vi "Game.vi"() -> ()   [LabVIEW 2012]
uses:
  <vilib>/Analysis/3filter.llb/Filter Passband Type.ctl
  Class/LV Wiimote Interface.lvclass
  <vilib>/ptbypt/NI_PtbyPt.lvlib
  <vilib>/Analysis/NI_AALBase.lvlib
panel:
  out "actual loop rate (ms)":u32
  in  "order":i32=2
  out "error":i32
  out "Waveform Chart":cluster{"X":sgl, "Filtered x":dbl}(graph)
  in  "low cutoff freq: fl":dbl=0.125 format="%0.3f"
  in  "Loop Rate":u32=50
  in  "high cutoff freq: fh":dbl=0.45000000000000007 format="%0.3f"
  in  "stop":bool
  in  "X, Y or Z":i32
  out "error out":errorcluster
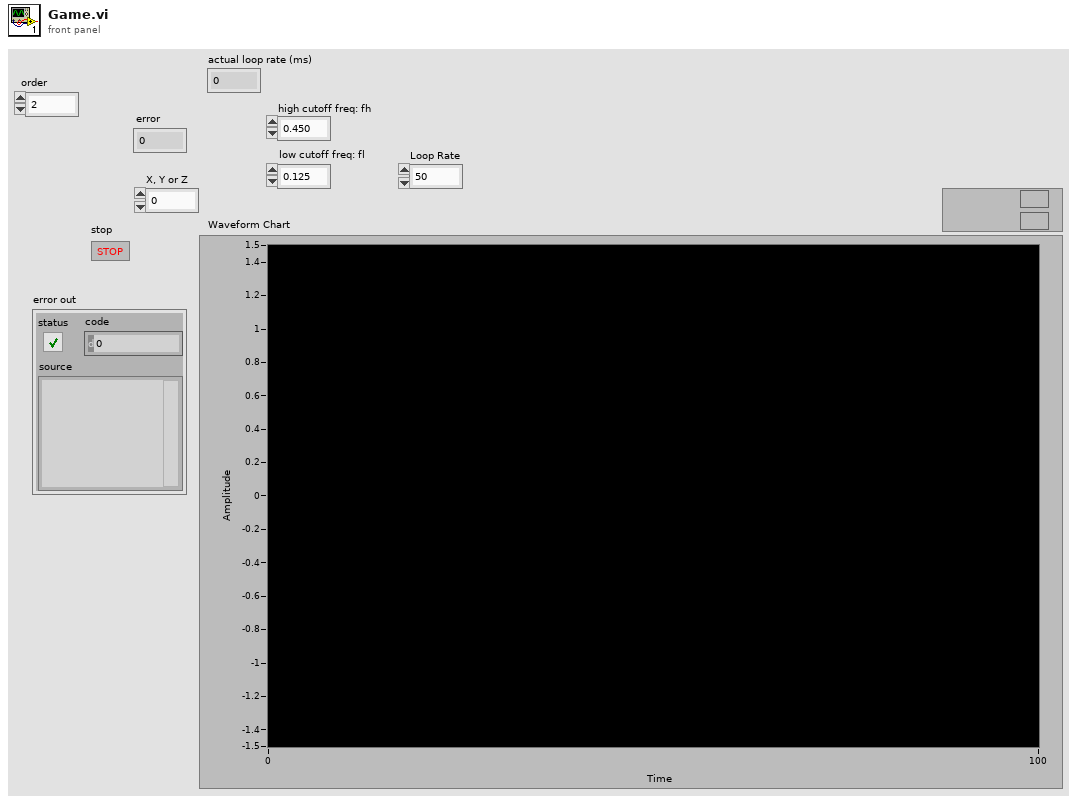
[diagram p1: front panel]
types:
  T1 = typedef "LV Wiimote Interface.ctl" = refnum<class "LV Wiimote Interface.lvclass">
  T2 = typedef "NI_AALBase.lvlib/Filter Passband Type.ctl" = enum32{"Lowpass", "Highpass", "Bandpass", "Bandstop"}
  T3 = typedef "LV Wiimote Interface.lvclass/XYZ Acceleration.ctl" = cluster{"X":sgl, "Y":sgl, "Z":sgl}
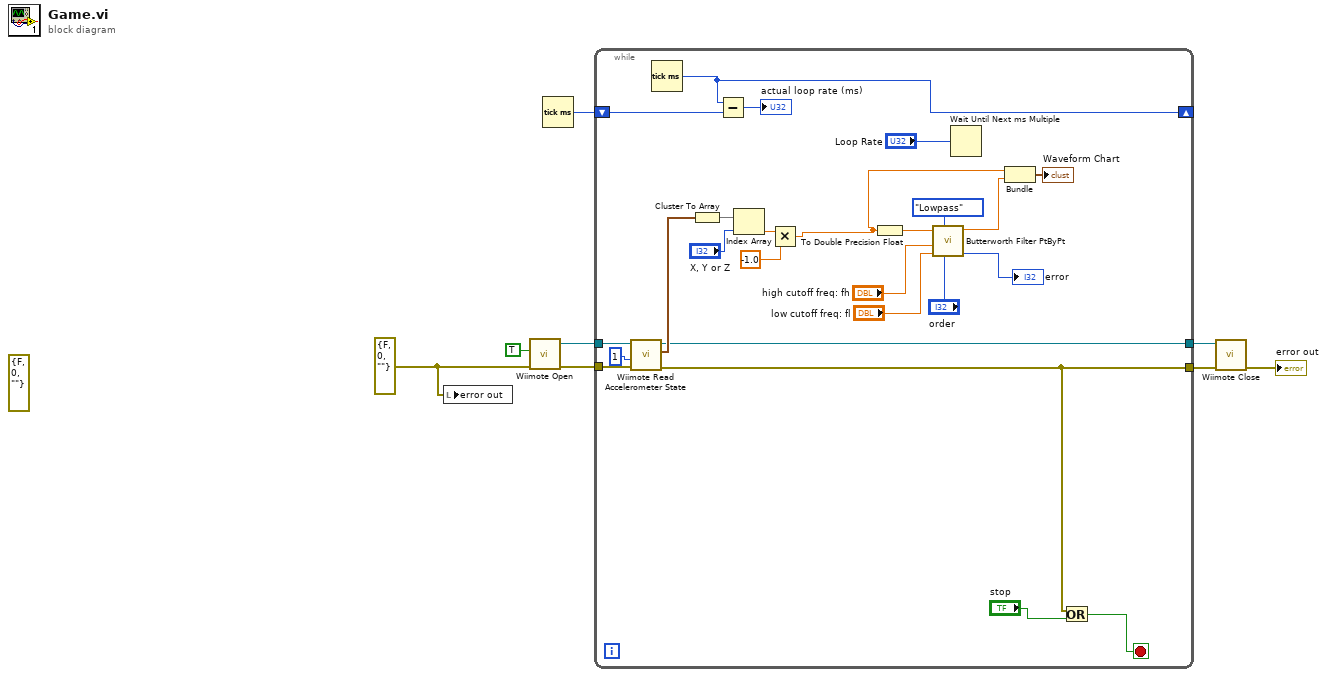
[diagram p0: block diagram]
diagram:
  w7 = errorcluster {"status"=FALSE, "code"=0, "source"=""} ("error in (no error)")
  (unwired) errorcluster {"status"=FALSE, "code"=0, "source"=""} ("error out")
  n1 = local write "error out"(w7) -> ()
  n2 = call "Wiimote Open.vi"("error in (no error)"=w7, "Connect to all?"=TRUE) -> ("error out"=w5:errorcluster, "LV WiiMote Interface"=w6:T1)  [unwired: 7 in, 1 out]
  n3 = Tick Count (ms)() -> (millisecond timer value=w1:u32)
  n4 = while {
    tunnel: w6 -> [w33]
    tunnel: w5 -> [w32]
    tunnel: [w27] -> w4
    tunnel: [w25] -> w3
    shift-right: [w13] -> _
    shift-left: w1 -> [w14]
    stop <- w26 stop-if-true
    n5 = call "Wiimote Read Accelerometer State.vi"("error in (no error)"=w32, "Wiimote Player #"=1, "LV WiiMote Interface In"=w33) -> ("error out"=w25:errorcluster, "XYZ Acceleration"=w30:T3, "LV WiiMote Interface out"=w27:T1)  [unwired: 6 in]
    n6 = Tick Count (ms)() -> (millisecond timer value=w13:u32)
    n7 = Cluster To Array(cluster=w30) -> (array=w29:sgl[])
    n8 = Subtract(x=w13, y=w14) -> (x-y=→"actual loop rate (ms)":u32)
    n9 = Index Array(array=w29, index="X, Y or Z") -> (element=w11:sgl)
    n10 = Multiply(x=w11, y=sgl -1.0) -> (x*y=w9:sgl)
    n11 = To Double Precision Float(number=w9) -> (double precision float=w23:dbl)
    n12 = call <vilib>:"Butterworth Filter PtByPt.vi"("order"="order", "filter type"=Filter_Passband_Type."Lowpass", "low cutoff freq: fl"="low cutoff freq: fl", "high cutoff freq: fh"="high cutoff freq: fh", "x"=w23) -> ("error"=→"error":i32, "Filtered x"=w17:dbl)  [unwired: 4 in]
    n13 = Wait Until Next ms Multiple(millisecond multiple="Loop Rate") -> ()  [unwired: 1 out]
    n14 = Bundle(w9, "Filtered x"=w17) -> (→"Waveform Chart":cluster{sgl, "Filtered x":dbl})  [unwired: 1 in]
    n15 = Or(x=w25, y="stop") -> (x .or. y?=w26:bool)
  }
  n16 = call "Wiimote Close.vi"("error in (no error)"=w3, "LV WiiMote Interface"=w4) -> ("error out"=→"error out":errorcluster)  [unwired: 9 in]
